vi "multuple ROI lines.vi"(8 "Width":u32=1, 9 "line color":u32(colorbox)=16711680, 10 "ROI":T2, 11 "Image in":T1) -> (3 "Image out":T1)   [LabVIEW 2012]
uses:
  <vilib>/vision/Image Controls.llb/IMAQ Image.ctl
panel:
  out "error out":errorcluster
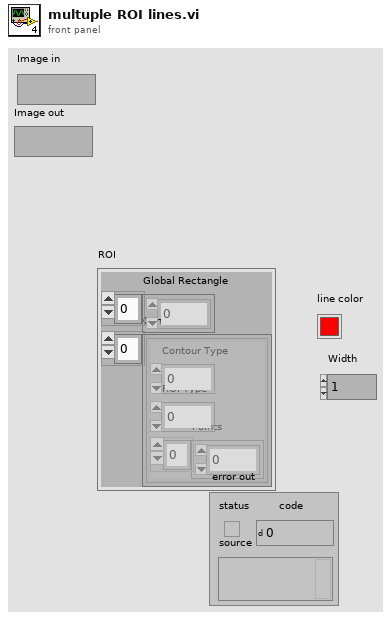
[diagram p1: front panel]
types:
  T1 = typedef "IMAQ Image.ctl" = refnum<image>
  T2 = cluster{"Global Rectangle":i32[], "Contours":cluster{"Contour Type":u32, "ROI Type":u32, "Points":i32[]}[]}
  T3 = cluster{"Contour Type":u32, "ROI Type":u32, "Points":i32[]}[]
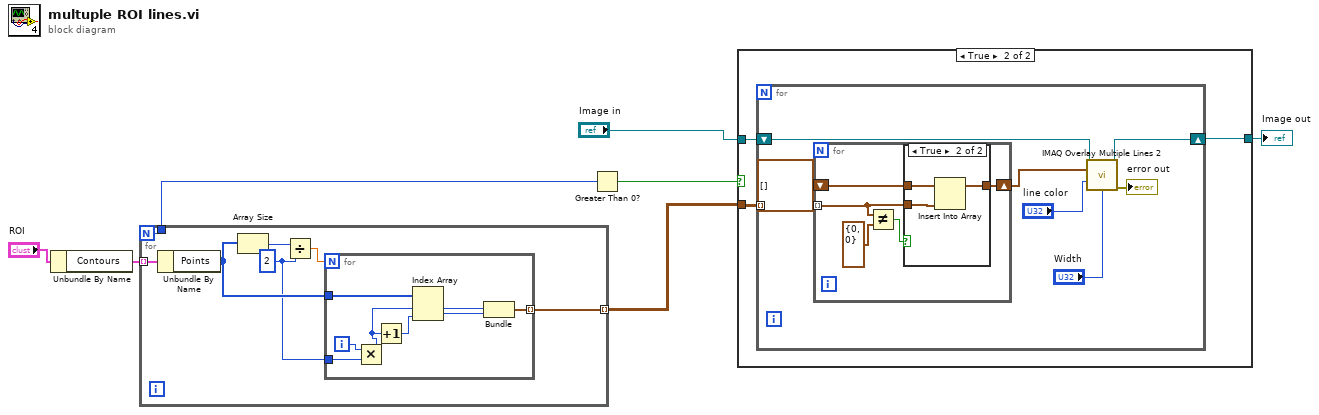
[diagram p0: block diagram]
diagram:
  n1 = Unbundle By Name("ROI") -> ("Contours"=w7:T3)
  n2 = for {
    N -> [w8]
    tunnel: w7 -> [w14] mode=indexing
    tunnel: [w10] -> w3 mode=indexing
    tunnel: [w8] -> w5
    w9 = 2 ("y")
    n3 = Unbundle By Name(w14) -> ("Points"=w13:i32[])
    n4 = Array Size(array=w13) -> (size(s)=w12:i32)
    n5 = Divide(x=w12, y=w9) -> (x/y=w11:dbl)
    n6 = for {
      N: w11 -> [_]
      tunnel: w13 -> [w22]
      tunnel: [w20] -> w10 mode=indexing
      tunnel: w9 -> [w16]
      i -> [w17]
      n7 = Multiply(x=w17, y=w16) -> (x*y=w15:i32)
      n8 = Increment(x=w15) -> (x+1=w21:i32)
      n9 = Index Array(array=w22, index #1=w15, index #2=w21) -> (element #1=w19:i32, element #2=w18:i32)
      n10 = Bundle(w19, w18) -> (w20:cluster{i32, i32})  [unwired: 1 in]
    }
  }
  n11 = Greater Than 0?(x=w5) -> (x > 0?=w4:bool)
  n12 = case shown="True" w4 {
    tunnel: "Image in" -> [w23 w26]
    tunnel: [w23 w25] -> w1
    tunnel: w3 -> [_ w24]
    frame False {
    }
    frame True {
      n13 = for {
        shift-right: [w33] -> w25
        shift-left: w26 -> [w34]
        tunnel: w24 -> [w30] mode=indexing
        n14 = for {
          tunnel: w30 -> [w37] mode=indexing
          shift-right: [w36] -> w29
          shift-left: cluster{i32, i32}[] [] -> [w35]
          n15 = Not Equal?(x=w37, y=cluster{i32, i32} {0, 0}) -> (x != y?=w38:bool)
          n16 = case shown="True" w38 {
            tunnel: w37 -> [_ w43]
            tunnel: [w40 w42] -> w36
            tunnel: w35 -> [w40 w41]
            frame False {
            }
            frame True {
              n17 = Insert Into Array(array=w41, new element=w43) -> (w42:cluster{i32, i32}[])  [unwired: 1 in]
            }
          }
        }
        n18 = call "IMAQ Overlay Multiple Lines 2"("Image"=w34, "Line End Points"=w29, "Color"="line color", "Width"="Width") -> ("Image Out"=w33:T1, "error out"=→"error out":errorcluster)  [unwired: 10 in]
      }
    }
  }
  "Image out" <- w1
